vi "Configure Jitter Spectrum (Phase).vi"(0 "VISA resource name":refnum<visa-resource-name>, 1 "Enable Jitter Spectrum (Enable)":bool, 5 "Source 1 (1: Channel 1)":i32(ring) items=["Channel 1", "Channel 2", "Channel 3", "Channel 4", "Function 1", "Function 2", "Function 3", "Function 4", "Memory 1", "Memory 2", "Memory 3", "Memory 4"], 7 "Source 2 (2: Channel 2)":i32(ring) items=["Channel 1", "Channel 2", "Channel 3", "Channel 4", "Function 1", "Function 2", "Function 3", "Function 4", "Memory 1", "Memory 2", "Memory 3", "Memory 4"], 9 "Direction (0: Rising)":i32(ring) items=["Rising", "Falling"], 11 "error in (no error)":errorcluster) -> (4 "VISA resource name out":refnum<visa-resource-name>, 15 "error out":errorcluster)   [LabVIEW 2009, in "Agilent 8000 Series.lvlib"]
doc: "Configures the Phase measurement and enables the Jitter Spectrum Jitter analysis on it.\n\n<B>Note:</B>\nCalling this VI disables all previously enabled measurements and clears existing measurement results from display."
uses:
  Agilent 8000 Series.lvlib
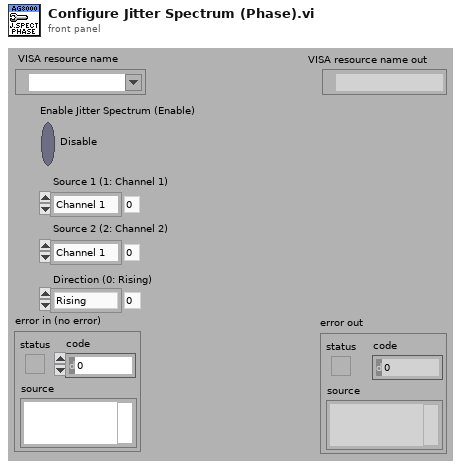
[diagram p1: front panel]
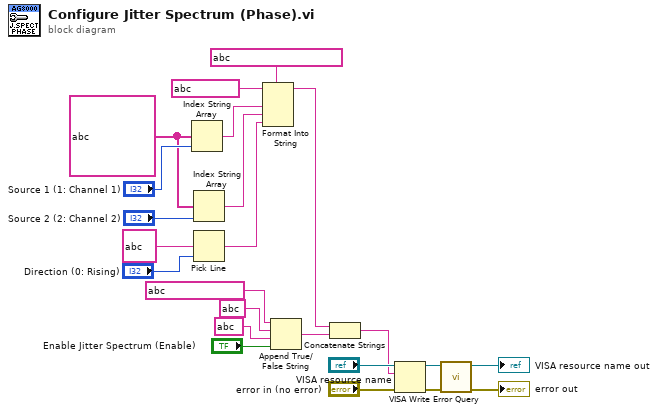
[diagram p0: block diagram]
diagram:
  w11 = string[] ?
  n1 = Index String Array(1:"Source 1 (1: Channel 1)", 2:w11) -> (0:w13:string)  [unwired: 1 in]
  n2 = Index String Array(1:"Source 2 (2: Channel 2)", 2:w11) -> (0:w10:string)  [unwired: 1 in]
  n3 = Pick Line(multi-line string=string ?, line index="Direction (0: Rising)") -> (output string=w8:string)  [unwired: 1 in]
  n4 = Format Into String(format string=string ?, initial string=string ?, w13, w10, w8) -> (resulting string=w3:string)  [unwired: 1 in, 1 out]
  n5 = Append True/False String(1:"Enable Jitter Spectrum (Enable)", 2:string ? ("false string"), 3:string ? ("true string"), 4:string ? ("string (\"\")")) -> (0:w2:string)
  n6 = Concatenate Strings(w3, w2) -> (w1:string)
  n7 = VISA Write(VISA resource name="VISA resource name", write buffer=w1, error in (no error)="error in (no error)") -> (VISA resource name out=w19:refnum<visa-resource-name>, error out=w18:errorcluster)  [unwired: 1 out]
  n8 = call "Error Query.vi"("error in (no error)"=w18, "VISA resource name"=w19) -> ("error out"=→"error out":errorcluster, "VISA resource name out"=→"VISA resource name out":refnum<visa-resource-name>)  [unwired: 6 in, 2 out]
